vi "Programm beenden.vi"() -> ()   [LabVIEW 2020, in "allgemeine Sub-VIs.lvlib"]
uses:
  allgemeine Sub-VIs.lvlib
  IAG-Logo-Auto B02.ctl
panel:
  in  "IAG":T1
  out "Schieberegler":u8(slide) scale=0.0..100.0
  out "String 2":string
  out "String":string
  out "Fehler":bool
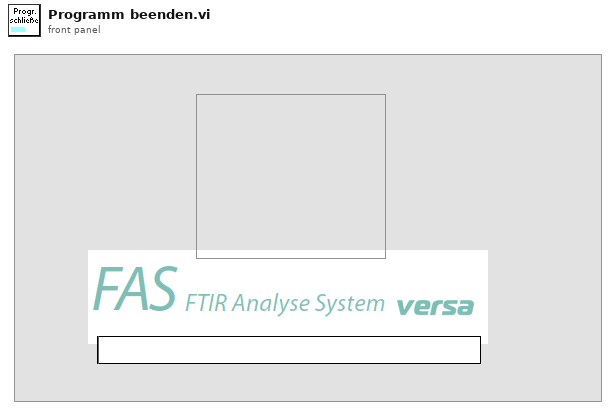
[diagram p1: front panel]
types:
  T1 = typedef "IAG-Logo-Auto B02.ctl" = bool
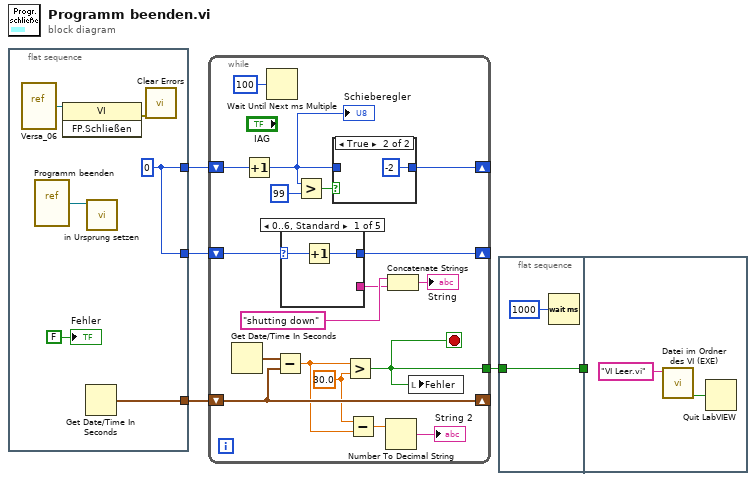
[diagram p0: block diagram]
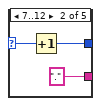
[diagram p2: hidden frame]
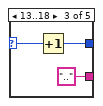
[diagram p3: hidden frame]
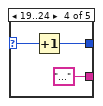
[diagram p4: hidden frame]
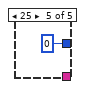
[diagram p5: hidden frame]
diagram:
  n1 = flat-sequence {
    tunnel: [w11] -> w5
    tunnel: [w11] -> w4
    tunnel: [w7] -> w3
    frame #0 {
      w11 = i8 0 ("Schieberegler")
      n2 = vi-ref "Versa_06.vi"() -> (w9:refnum<vi>)
      n3 = vi-ref "Programm beenden.vi"() -> (w10:refnum<vi>)
      n4 = invoke class="VI" method="FP.Schließen"(reference=w9) -> (error out=w8:errorcluster)  [unwired: 2 in, 2 out]
      n5 = Get Date/Time In Seconds() -> (seconds since 1Jan1904=w7:timestamp)
      n6 = call "in Ursprung setzen.vi"("VI Referenz"=w10) -> ()  [unwired: 10 in, 1 out]
      n7 = call <vilib>:"Clear Errors.vi"("error in (no error)"=w8) -> ()  [unwired: 5 in, 2 out]
      "Fehler" <- FALSE ("Fehler")
    }
  }
  n8 = while {
    shift-right: [w27] -> _
    shift-left: w5 -> [w25]
    shift-right: [w23] -> _
    shift-left: w4 -> [w24]
    shift-right: [w17] -> _
    shift-left: w3 -> [w17]
    tunnel: [w16] -> w2
    stop <- w16 stop-if-true
    w15 = 30.0 ("y")
    n9 = Get Date/Time In Seconds() -> (seconds since 1Jan1904=w18:timestamp)
    n10 = Increment(x=w25) -> (x+1=w19:i8)
    "Schieberegler" <- w19
    n11 = Wait Until Next ms Multiple(millisecond multiple=u32 100 ("Vielfache von ms")) -> ()  [unwired: 1 out]
    n12 = Subtract(x=w18, y=w17) -> (x-y=w14:dbl)
    n13 = case shown="0..6, Standard" w24 {
      selector: w24 -> [w31 w34 w36 w40 _]
      tunnel: [w30 w33 w37 w39 i8 0] -> w23
      tunnel: [_ "." ".." "..." _] -> w21
      frame 0..6, Default {
        n14 = Increment(x=w31) -> (x+1=w30:i8)
      }
      frame 7..12 {
        n15 = Increment(x=w34) -> (x+1=w33:i8)
      }
      frame 13..18 {
        n16 = Increment(x=w36) -> (x+1=w37:i8)
      }
      frame 19..24 {
        n17 = Increment(x=w40) -> (x+1=w39:i8)
      }
      frame 25 {
      }
    }
    n18 = Greater?(x=w19, y=i8 99) -> (0:w28:bool)
    n19 = case shown="True" w28 {
      tunnel: w19 -> [w42 _]
      tunnel: [w42 i8 -2] -> w27
      frame False {
      }
      frame True {
      }
    }
    n20 = Greater?(x=w14, y=w15) -> (0:w16:bool)
    n21 = Subtract(x=w15, y=w14) -> (x-y=w13:dbl)
    n22 = Number To Decimal String(number=w13) -> (decimal integer string=→"String 2":string)  [unwired: 1 in]
    n23 = Concatenate Strings("shutting down" ("String"), w21) -> (→"String":string)
    n24 = local write "Fehler"(w16) -> ()
  }
  n25 = flat-sequence {
    tunnel: w2 -> [w45]
    tunnel: [w45] -> w1
    tunnel: w1 -> [_]
    frame #0 {
      n26 = Wait (ms)(milliseconds to wait=u32 1000 ("Zu wartende ms")) -> ()  [unwired: 1 out]
    }
    frame #1 {
      n27 = call "Datei im Ordner des VI (EXE).vi"("Dateiname"="VI Leer.vi") -> ("EXE"=w46:bool)  [unwired: 8 in, 2 out]
      n28 = Quit LabVIEW(quit? (T)=w46) -> ()
    }
  }
